vi "DSF.Engine.Memory.Pointer.VS Channels.Get Channel Count.vi"(8 "error in (no error)":errorcluster, 11 "VS Channels Pointer in":refnum<class "DSF.Engine.Memory.Pointer.VS Channels.lvclass">) -> (0 "error out":errorcluster, 2 "channel count":u64 format="%d channels", 3 "VS Channels Pointer out":refnum<class "DSF.Engine.Memory.Pointer.VS Channels.lvclass">)   [LabVIEW 2016, in "DSF.Engine.lvlib" / "DSF.Engine.Memory.Pointer.VS Channels.lvclass"]
uses:
  DSF.Engine.Memory.Pointer.VS Channels.lvclass
  DSF.Engine.Memory.Pointer.VS Channels.lvclass/DSF.Engine.Memory.Pointer.VS Channels.ctl
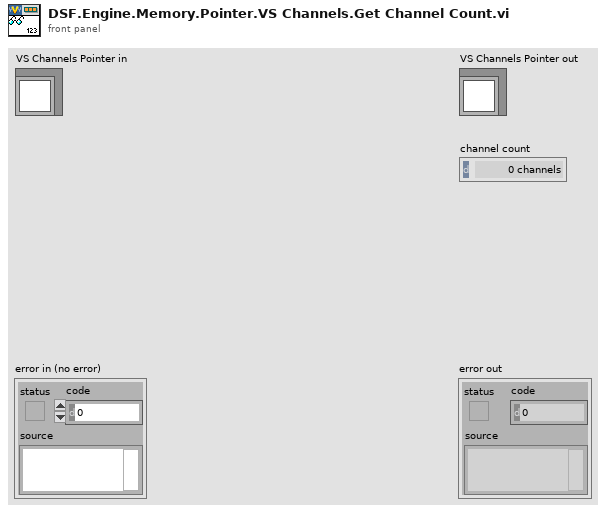
[diagram p1: front panel]
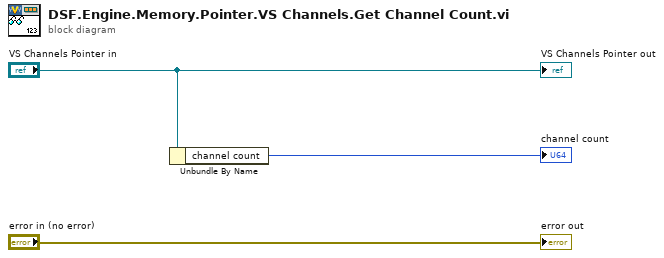
[diagram p0: block diagram]
diagram:
  n1 = Unbundle By Name("VS Channels Pointer in") -> ("channel count"=→"channel count":u64)
  "error out" <- "error in (no error)"
  "VS Channels Pointer out" <- "VS Channels Pointer in"
